vi "default cluster.vi"(11 "size":i32) -> (3 "Array":T1(array[cluster]) {"Kelvin Yk-1" format="%.4p"; "1R Yk-1" format="%.4p"; "10R Yk-1" format="%.4p"; "Wagner Yk-1" format="%.4p"; "Ana Denge Yk-1" format="%.4p"; "Kelvin Yk" format="%.4p"; "1R Yk" format="%.4p"; "10R Yk" format="%.4p"; "Wagner Yk" format="%.4p"; "Ana Denge Yk" format="%.4p"; "Kelvin Xk-1" format="%.4p"; "1R Xk-1" format="%.4p"; "10R Xk-1" format="%.4p"; "Wagner Xk-1" format="%.4p"; "Ana Denge Xk-1" format="%.4p"; "Kelvin Xk" format="%.4p"; "1R Xk" format="%.4p"; "10R Xk" format="%.4p"; "Wagner Xk" format="%.4p"; "Ana Denge Xk" format="%.4p"})   [LabVIEW 2014]
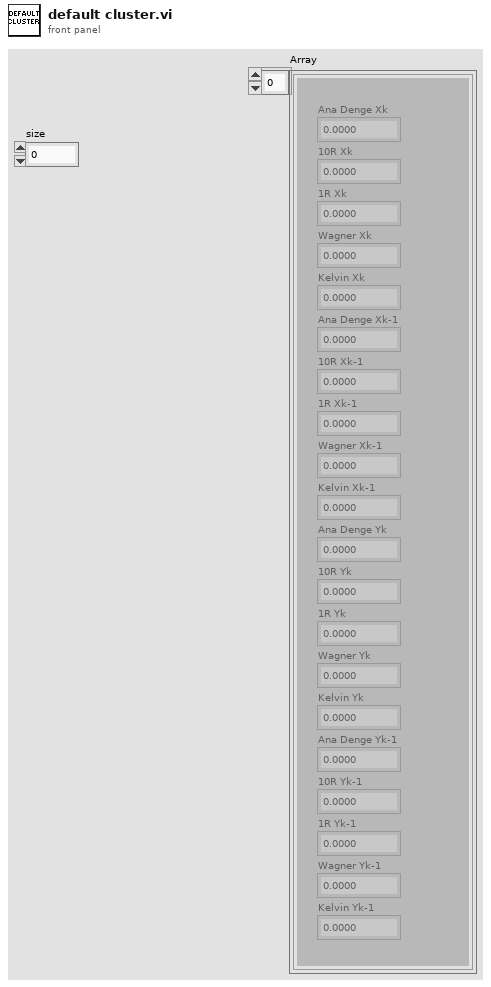
[diagram p1: front panel]
types:
  T1 = cluster{"Ana Denge Xk":dbl, "Wagner Xk":dbl, "10R Xk":dbl, "1R Xk":dbl, "Kelvin Xk":dbl, "Ana Denge Xk-1":dbl, "Wagner Xk-1":dbl, "10R Xk-1":dbl, "1R Xk-1":dbl, "Kelvin Xk-1":dbl, "Ana Denge Yk":dbl, "Wagner Yk":dbl, "10R Yk":dbl, "1R Yk":dbl, "Kelvin Yk":dbl, "Ana Denge Yk-1":dbl, "Wagner Yk-1":dbl, "10R Yk-1":dbl, "1R Yk-1":dbl, "Kelvin Yk-1":dbl}[]
  T2 = cluster{"Ana Denge Xk":dbl, "Wagner Xk":dbl, "10R Xk":dbl, "1R Xk":dbl, "Kelvin Xk":dbl, "Ana Denge Xk-1":dbl, "Wagner Xk-1":dbl, "10R Xk-1":dbl, "1R Xk-1":dbl, "Kelvin Xk-1":dbl, "Ana Denge Yk":dbl, "Wagner Yk":dbl, "10R Yk":dbl, "1R Yk":dbl, "Kelvin Yk":dbl, "Ana Denge Yk-1":dbl, "Wagner Yk-1":dbl, "10R Yk-1":dbl, "1R Yk-1":dbl, "Kelvin Yk-1":dbl}
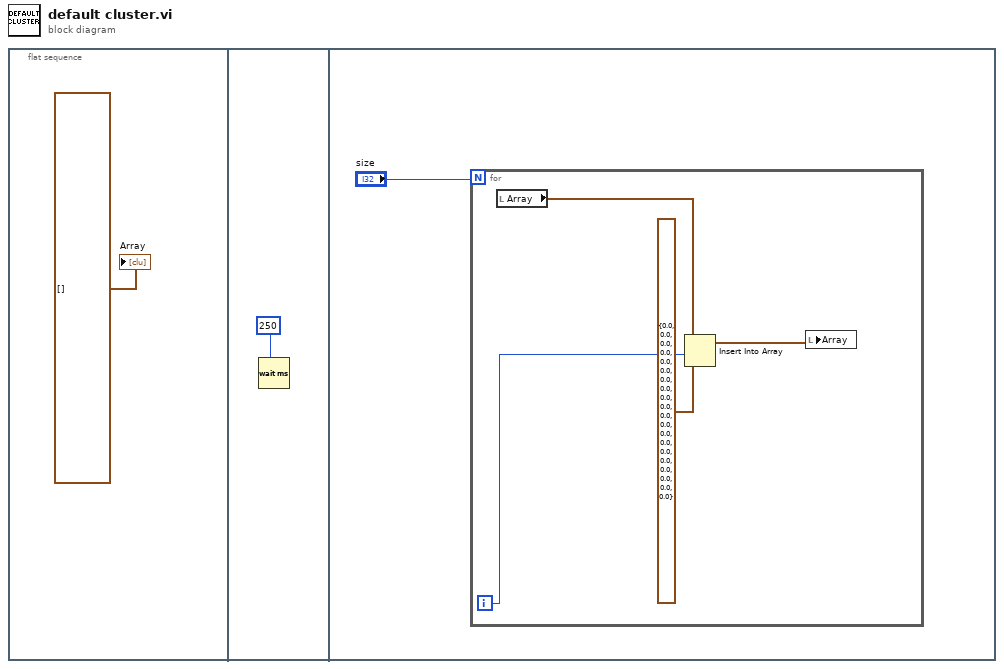
[diagram p0: block diagram]
diagram:
  n1 = flat-sequence {
    frame #0 {
      "Array" <- T1 [] ("Array")
    }
    frame #1 {
      n2 = Wait (ms)(milliseconds to wait=u32 250) -> ()  [unwired: 1 out]
    }
    frame #2 {
      n3 = for {
        N: "size" -> [_]
        i -> [w6]
        n4 = local read "Array"() -> (w4:T1)
        n5 = Insert Into Array(array=w4, index=w6, new element=T2 {"Ana Denge Xk"=0.0, "Wagner Xk"=0.0, "10R Xk"=0.0, "1R Xk"=0.0, "Kelvin Xk"=0.0, "Ana Denge Xk-1"=0.0, "Wagner Xk-1"=0.0, "10R Xk-1"=0.0, "1R Xk-1"=0.0, "Kelvin Xk-1"=0.0, "Ana Denge Yk"=0.0, "Wagner Yk"=0.0, "10R Yk"=0.0, "1R Yk"=0.0, "Kelvin Yk"=0.0, "Ana Denge Yk-1"=0.0, "Wagner Yk-1"=0.0, "10R Yk-1"=0.0, "1R Yk-1"=0.0, "Kelvin Yk-1"=0.0} ("new element/subarray")) -> (w7:T1)
        n6 = local write "Array"(w7) -> ()
      }
    }
  }
